vi "Intake Ramp (2).vi"(10 "Intake":bool, 11 "Outtake":bool) -> ()   [LabVIEW 2016]
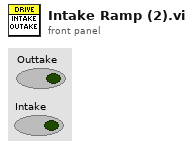
[diagram p1: front panel]
types:
  T1 = typedef "WPI_MotorControlDeviceRef.ctl" = cluster{"DeviceStatus":errorcluster, "Type":T2, "PWM":cluster{"PWM Channel":T3, "DeadBand":T4}, "CAN":cluster{"Device Number":u8, "SetOutput VI Ref":variant, "GetOutput VI Ref":variant, "Enable VI Ref":variant, "Disable VI Ref":variant, "Data":variant}, "Invert":bool}
  T2 = typedef "WPI_MotorControlType.ctl" = enum16{"PWM", "CAN"}
  T3 = typedef "FPGA_DIOPWMChannel.ctl" = enum8{"PWM 0", "PWM 1", "PWM 2", "PWM 3", "PWM 4", "PWM 5", "PWM 6", "PWM 7", "PWM 8", "PWM 9", "PWM MXP 0", "PWM MXP 1", "PWM MXP 2", "PWM MXP 3", "PWM MXP 4", "PWM MXP 5", "PWM MXP 6", "PWM MXP 7", "PWM MXP 8", "PWM MXP 9", "Invalid"}
  T4 = typedef "WPI_PWMDeadband.ctl" = cluster{"Name":string, "maxPositivePwm":i32, "minPositivePwm":i32, "centerPwm":i32, "maxNegativePwm":i32, "minNegativePwm":i32, "angularRange":u16}
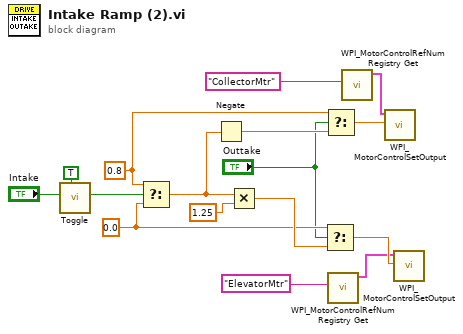
[diagram p0: block diagram]
diagram:
  w9 = 0.8 ("t")
  w8 = 0.0 ("f")
  n1 = call "Toggle.vi"("Control"=TRUE, "Input"="Intake") -> ("Output"=w16:bool)  [unwired: 9 in]
  n2 = Select(t=w9, s=w16, f=w8) -> (s? t:f=w14:dbl)
  n3 = Negate(x=w14) -> (-x=w13:dbl)
  n4 = Multiply(x=w14, y=1.25) -> (x*y=w12:dbl)
  n5 = Select(t=w8, s="Outtake", f=w12) -> (s? t:f=w10:dbl)
  n6 = Select(t=w9, s="Outtake", f=w13) -> (s? t:f=w11:dbl)
  n7 = call <vilib>:"WPI_MotorControlRefNum Registry Get.vi"("refnum name"="ElevatorMtr") -> ("MotorControlDevRef"=w5:T1)  [unwired: 9 in, 1 out]
  n8 = call <vilib>:"WPI_MotorControlRefNum Registry Get.vi"("refnum name"="CollectorMtr") -> ("MotorControlDevRef"=w3:T1)  [unwired: 9 in, 1 out]
  n9 = call <vilib>:"WPI_MotorControlSetOutput.vi"("Output"=w11, "MotorControlDevRef"=w3) -> ()  [unwired: 7 in, 3 out]
  n10 = call <vilib>:"WPI_MotorControlSetOutput.vi"("Output"=w10, "MotorControlDevRef"=w5) -> ()  [unwired: 7 in, 3 out]
